vi "Overlay 直線兩端點.vi"(5 "size":dbl=10.0, 6 "Color 2":u32(colorbox)=16711680, 7 "Group":string, 8 "error in":errorcluster, 9 "Arrows":cluster{"Start point":bool, "End point":bool}, 10 "Line Coordinates":T2, 11 "Image In":T1) -> (0 "error out 2":errorcluster, 3 "Image Out 2":T1)   [LabVIEW 2015]
uses:
  <vilib>/vision/Image Controls.llb/IMAQ Image.ctl
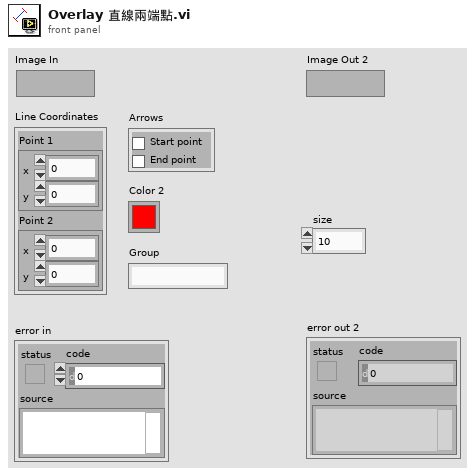
[diagram p1: front panel]
types:
  T1 = typedef "IMAQ Image.ctl" = refnum<image>
  T2 = cluster{"Point 1":cluster{"x":dbl, "y":dbl}, "Point 2":cluster{"x":dbl, "y":dbl}}
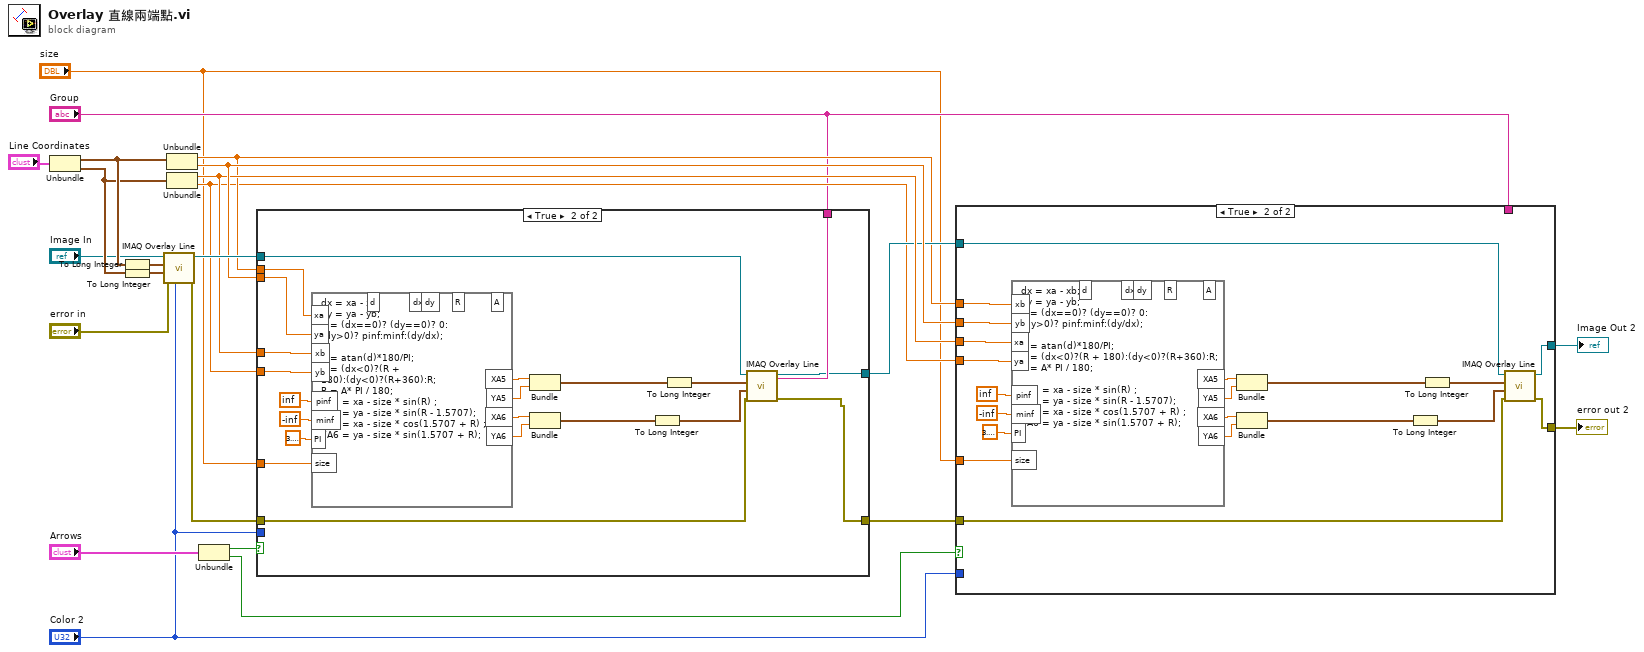
[diagram p0: block diagram]
diagram:
  n1 = Unbundle("Line Coordinates") -> ("Point 1"=w15:cluster{"x":dbl, "y":dbl}, "Point 2"=w14:cluster{"x":dbl, "y":dbl})
  n2 = To Long Integer(number=w15) -> (32bit integer=w13:cluster{"x":i32, "y":i32})
  n3 = To Long Integer(number=w14) -> (32bit integer=w12:cluster{"x":i32, "y":i32})
  n4 = call "IMAQ Overlay Line"("Color"="Color 2", "error in (no error)"="error in", "End Point"=w12, "Start Point"=w13, "Image"="Image In") -> ("error out"=w8:errorcluster, "Image Out"=w23:T1)  [unwired: 1 in, 4 out]
  n5 = Unbundle(w15) -> ("x"=w11:dbl, "y"=w21:dbl)
  n6 = Unbundle(w14) -> ("x"=w20:dbl, "y"=w10:dbl)
  n7 = Unbundle("Arrows") -> ("Start point"=w18:bool, "End point"=w2:bool)
  n8 = case shown="True" w18 {
    tunnel: w11 -> [_ w38]
    tunnel: w21 -> [_ w37]
    tunnel: w20 -> [_ w39]
    tunnel: w10 -> [_ w36]
    tunnel: w23 -> [w25 w30]
    tunnel: [w25 w27] -> w16
    tunnel: "Color 2" -> [_ _]
    tunnel: w8 -> [w24 w28]
    tunnel: [w24 w26] -> w7
    tunnel: "Group" -> [_ w29]
    tunnel: "size" -> [_ w35]
    frame False {
    }
    frame True {
      n9 = formula code="dx = xa - xb;\ndy = ya - yb;\nd = (dx==0)? (dy==0)? 0: \n(dy>0)? pinf:minf:(dy/dx);\n\nR = atan(d)*180/PI;\nA = (dx<0)?(R + 180):(dy<0)?(R+360):R;\nR = A* PI / 180;\nXA5 = xa - size * sin(R) ;\nYA5 = ya - size * sin(R - 1.5707);\nXA6 = xa - size * cos(1.5707 + R) ;\nYA6 = ya - size * sin(1.5707 + R);"("xa"=w38, "ya"=w37, "xb"=w39, "yb"=w36, "pinf"=inf, "minf"=-inf, "PI"=3.141592653589793, "size"=w35) -> ("XA5"=w43:dbl, "YA5"=w42:dbl, "XA6"=w41:dbl, "YA6"=w40:dbl)  [unwired: 5 out]
      n10 = Bundle("XA5"=w43, "YA5"=w42) -> (w34:cluster{"XA5":dbl, "YA5":dbl})  [unwired: 1 out]
      n11 = Bundle("XA6"=w41, "YA6"=w40) -> (w32:cluster{"XA6":dbl, "YA6":dbl})  [unwired: 1 out]
      n12 = To Long Integer(number=w32) -> (32bit integer=w31:cluster{"XA6":i32, "YA6":i32})
      n13 = To Long Integer(number=w34) -> (32bit integer=w33:cluster{"XA5":i32, "YA5":i32})
      n14 = call "IMAQ Overlay Line"("Group"=w29, "error in (no error)"=w28, "End Point"=w31, "Start Point"=w33, "Image"=w30) -> ("error out"=w26:errorcluster, "Image Out"=w27:T1)  [unwired: 1 in, 4 out]
    }
  }
  n15 = case shown="True" w2 {
    tunnel: w11 -> [_ w65]
    tunnel: w21 -> [_ w64]
    tunnel: w20 -> [_ w63]
    tunnel: w10 -> [_ w62]
    tunnel: w16 -> [w48 w51]
    tunnel: [w48 w52] -> w17
    tunnel: "Color 2" -> [_ _]
    tunnel: w7 -> [w47 w50]
    tunnel: [w47 w49] -> w6
    tunnel: "Group" -> [_ _]
    tunnel: "size" -> [_ w57]
    frame False {
    }
    frame True {
      n16 = formula code="dx = xa - xb;\ndy = ya - yb;\nd = (dx==0)? (dy==0)? 0:\n(dy>0)? pinf:minf:(dy/dx);\n\nR = atan(d)*180/PI;\nA = (dx<0)?(R + 180):(dy<0)?(R+360):R;\nR = A* PI / 180;\n\nXA5 = xa - size * sin(R) ;\nYA5 = ya - size * sin(R - 1.5707);\nXA6 = xa - size * cos(1.5707 + R) ;\nYA6 = ya - size * sin(1.5707 + R);"("xb"=w65, "yb"=w64, "xa"=w63, "ya"=w62, "pinf"=inf, "minf"=-inf, "PI"=3.141592653589793, "size"=w57) -> ("XA5"=w61:dbl, "YA5"=w60:dbl, "XA6"=w59:dbl, "YA6"=w58:dbl)  [unwired: 5 out]
      n17 = Bundle("XA5"=w61, "YA5"=w60) -> (w54:cluster{"XA5":dbl, "YA5":dbl})  [unwired: 1 out]
      n18 = Bundle("XA6"=w59, "YA6"=w58) -> (w53:cluster{"XA6":dbl, "YA6":dbl})  [unwired: 1 out]
      n19 = To Long Integer(number=w53) -> (32bit integer=w55:cluster{"XA6":i32, "YA6":i32})
      n20 = To Long Integer(number=w54) -> (32bit integer=w56:cluster{"XA5":i32, "YA5":i32})
      n21 = call "IMAQ Overlay Line"("error in (no error)"=w50, "End Point"=w55, "Start Point"=w56, "Image"=w51) -> ("error out"=w49:errorcluster, "Image Out"=w52:T1)  [unwired: 2 in, 4 out]
    }
  }
  "Image Out 2" <- w17
  "error out 2" <- w6
